vi "Set WL Voltage.vi"(7 "Sample Rate":dbl=1000.0, 8 "error in (no error)":errorcluster) -> (0 "error out":errorcluster)   [LabVIEW 2019]
uses:
  <vilib>/DAQmx/write.llb/DAQmx Write (Analog 1D DBL NChan 1Samp).vi
  Globals.vi
  <vilib>/DAQmx/create/channels.llb/DAQmx Create Channel (AO-Voltage-Basic).vi
  <vilib>/DAQmx/configure/timing.llb/DAQmx Timing (Sample Clock).vi
  <vilib>/DAQmx/miscellaneous.llb/DAQmx Fill In Error Info.vi
panel:
  out "number of samples written per channel":u32
  out "AO0:3 Outputs (V)":dbl[](array[numeric])
  in  "VWL (V)":dbl
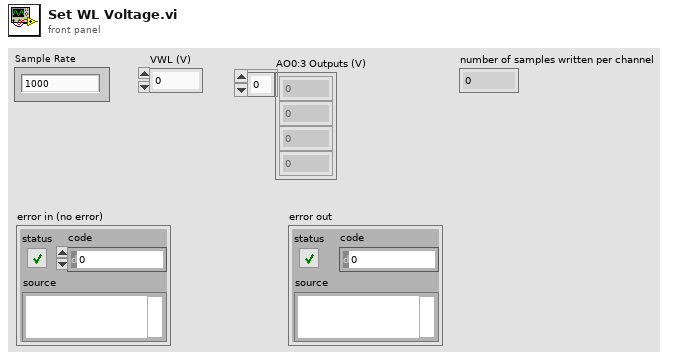
[diagram p1: front panel]
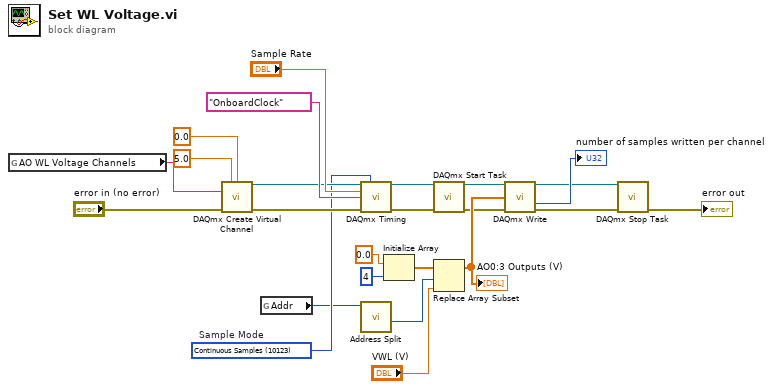
[diagram p0: block diagram]
diagram:
  w17 = 10123 items=["Finite Samples"=10178, "Continuous Samples"=10123, "Hardware Timed Single Point"=12522]  # Sample Mode
  n1 = global read "Globals.vi" "AO WL Voltage Channels"() -> (w9:tag)
  n2 = call-poly <vilib>:"DAQmx Create Virtual Channel.vi"("maximum value"=5.0 ("Max Voltage"), "minimum value"=0.0 ("Min Voltage"), "physical channels"=w9, "error in"="error in (no error)") -> ("task out"=w19:refnum<k21>, "error out"=w18:errorcluster)  [unwired: 10 in]
  n3 = global read "Globals.vi" "Addr"() -> (w16:u16)
  n4 = call-poly <vilib>:"DAQmx Timing.vi"("task/channels in"=w19, "sample mode"=w17, "rate"="Sample Rate", "source"=tag "OnboardClock" ("Sample Clock Source"), "error in"=w18) -> ("task out"=w8:refnum<k21>, "error out"=w7:errorcluster)  [unwired: 9 in]
  n5 = call "Address Split.vi"("address"=w16) -> ("wl_ext_sel"=w12:u32)  [unwired: 7 in, 3 out]
  n6 = Initialize Array(0.0 ("element"), 4 ("dimension size")) -> (w13:dbl[])
  n7 = call <vilib>:"DAQmx Start Task.vi"("task/channels in"=w8, "error in"=w7) -> ("task out"=w6:refnum<k21>, "error out"=w5:errorcluster)  [unwired: 12 in]
  n8 = Replace Array Subset(array=w13, new element="VWL (V)", index=w12) -> (w10:dbl[])
  "AO0:3 Outputs (V)" <- w10
  n9 = call-poly <vilib>:"DAQmx Write.vi"("task/channels in"=w6, "data"=w10, "error in"=w5) -> ("task out"=w3:refnum<k21>, "number of samples written per channel"=→"number of samples written per channel":u32, "error out"=w2:errorcluster)  [unwired: 10 in]
  n10 = call <vilib>:"DAQmx Stop Task.vi"("task/channels in"=w3, "error in"=w2) -> ("error out"=→"error out":errorcluster)  [unwired: 12 in, 1 out]
